vi "Test Barista Sends Pick Up Callback.vi"(8 "error in (no error)":errorcluster, 11 "Barista Test in":refnum<class "Barista Test.lvclass">) -> (0 "error out":errorcluster, 3 "Barista Test out":refnum<class "Barista Test.lvclass">)   [LabVIEW 2020, in "Barista Test.lvclass"]
uses:
  Barista Test.lvclass
  C:/Program Files (x86)/National Instruments/LabVIEW 2020/vi.lib/Astemes/LUnit/Test Case.lvclass
  Processes/People/Workers/Barista/Barista.lvclass
  C:/Program Files (x86)/National Instruments/LabVIEW 2020/vi.lib/Astemes/Triarc Framework/Process/Process.lvclass
  Support/Beverages/Beverage/Beverage.lvclass
  Test Doubles/Mock Job Handler/Mock Job Handler.lvclass
  C:/Git/astemes-triarc-examples/Coffee Shop/Processes/People/Process Job/Job Handler.lvclass
  Support/Beverages/TypeDefs/Drink Type.ctl
  Support/Beverages/TypeDefs/Options.ctl
  Support/Beverages/Beverage/Beverage.lvclass/Beverage.ctl
  <vilib>/Astemes/Triarc Framework/Process/Process.lvclass/Process.ctl
  <vilib>/Astemes/LUnit/Test Case.lvclass/Test Case.ctl
  89ef2f0c-66e7-4d1e-b839-78bb04362f4d.vi
  Support/Beverages/Beverage/Write Drink Type.vi
  Support/Beverages/Beverage/Write Options.vi
  <vilib>/Astemes/Triarc Framework/Process/Private/SubVIs/Wait for finish.vi
  <vilib>/Astemes/Triarc Framework/Process/Private/SubVIs/Set Lifecycle State.vi
  <vilib>/Astemes/Triarc Framework/Process/Protected/Messaging/Send Message.vi
  <vilib>/Astemes/Triarc Framework/Process/Public/Lifecycle/Get Lifecycle State.vi
  <vilib>/Astemes/LUnit/Palette/Pass.vi
  <vilib>/Astemes/LUnit/Palette/Fail.vi
  <vilib>/Astemes/LUnit/Compare Variants.vi
  <vilib>/Astemes/LUnit/Describe Comparison.vi
  <vilib>/Astemes/LUnit/Set Assertion Type.vi
  <vilib>/Astemes/Triarc Framework/Process/Private/SubVIs/Handle Debug Data.vi
  <vilib>/Utility/error.llb/Clear Errors.vi
  <vilib>/Astemes/LUnit/Add test result.vi
  <vilib>/Astemes/LUnit/Variant to string.vi
  <vilib>/Astemes/Triarc Framework/Logging/Log Debug.vi
  <vilib>/AdvancedString/1D String Array to Delimited String.vi
  <vilib>/Utility/High Resolution Relative Seconds.vi
  <vilib>/Astemes/LUnit/LUnit Record Assertion Result.vi
  <vilib>/Astemes/LUnit/LUnit Aggregate Assertion Results.vi
  <vilib>/Astemes/LUnit/Method Result/LUnit Merge Status.vi
  <vilib>/Astemes/LUnit/LUnit Concatenate result strings.vi
  <vilib>/Utility/error.llb/Error Cluster From Error Code.vi
  <vilib>/Astemes/Triarc Framework/Process/Public/Read Name.vi
  <vilib>/Utility/Data Type/Get Type Information.vi
  <vilib>/Utility/LVClass/Get LV Class Name.vi
  <vilib>/Astemes/Triarc Framework/Process/Process.lvclass
  Support/Order Item/Order Item.lvclass
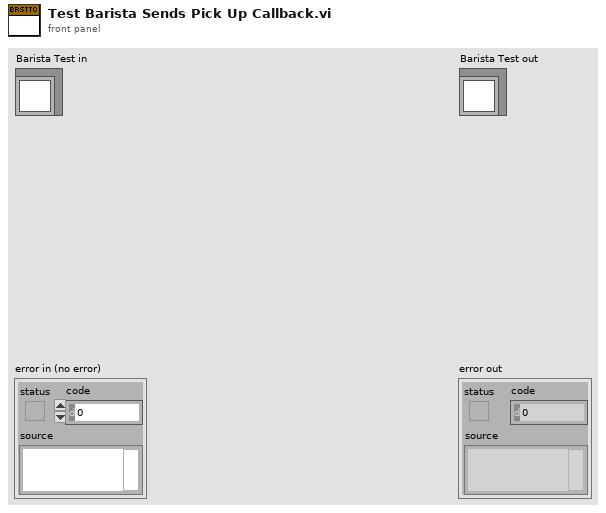
[diagram p1: front panel]
types:
  T1 = typedef "Beverage.lvclass/Options.ctl" = enum16{"<None>", "Milk", "Mocha", "Soy", "Whip"}
  T2 = typedef "Beverage.lvclass/Drink Type.ctl" = enum16{"Dark Roast", "Decaf", "Espresso", "House Blend"}
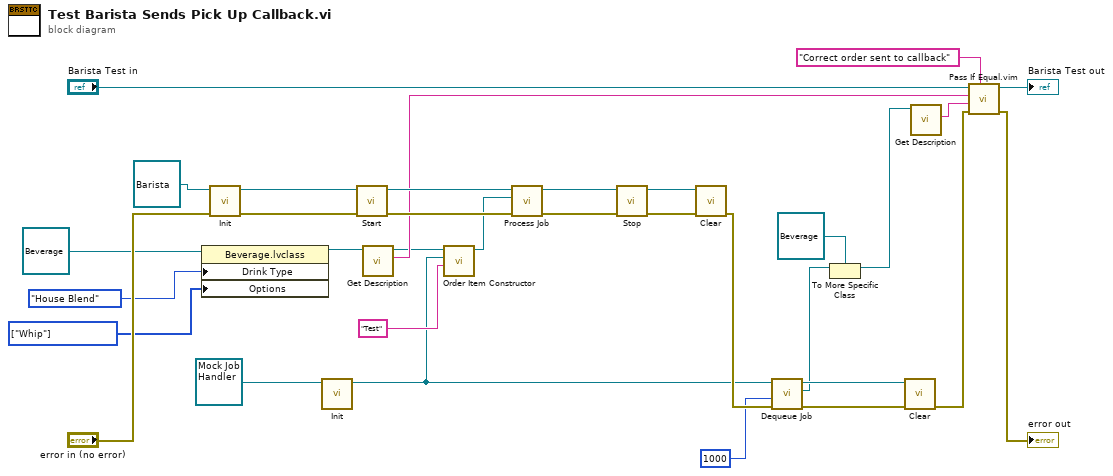
[diagram p0: block diagram]
diagram:
  w6 = T1[] [enum."Whip"] items=["<None>", "Milk", "Mocha", "Soy", "Whip"] ("Options")
  n1 = property class="Beverage.lvclass"(reference=refnum<class "Beverage.lvclass"> refnum ("Beverage"), "Drink Type"=Drink_Type."House Blend", "Options"=w6) -> (reference out=w5:refnum<class "Beverage.lvclass">)  [unwired: 1 in, 1 out]
  n2 = call-dynamic "Init.vi"("error in (no error)"="error in (no error)", "View In"=refnum<class "Barista.lvclass"> refnum ("Barista.lvclass")) -> ("error out"=w30:errorcluster, "View Out"=w26:refnum<class "Barista.lvclass">)  [unwired: 8 in]
  n3 = call-dynamic "Init.vi"("Mock Job Handler In"=refnum<class "Mock Job Handler.lvclass"> refnum ("Mock Job Handler.lvclass")) -> ("Mock Job Handler Out"=w9:refnum<class "Mock Job Handler.lvclass">)  [unwired: 9 in, 1 out]
  n4 = call <vilib>:"Start.vi"("error in (no error)"=w30, "Process In"=w26) -> ("error out"=w32:errorcluster, "Process Out"=w25:refnum<class "Barista.lvclass">)  [unwired: 7 in, 1 out]
  n5 = call "Get Description.vi"("Beverage in"=w5) -> ("Description"=w16:string, "Beverage out"=w4:refnum<class "Beverage.lvclass">)  [unwired: 8 in, 1 out]
  n6 = call "Order Item Constructor.vi"("Cust Name"="Test", "Pick Up Order Handler"=w9, "Beverage"=w4) -> ("Order Item"=w28:refnum<class "Order Item.lvclass">)  [unwired: 7 in, 1 out]
  n7 = call-dynamic "Process Job.vi"("error in (no error)"=w32, "Job"=w28, "Worker In"=w25) -> ("error out"=w22:errorcluster, "Worker Out"=w24:refnum<class "Barista.lvclass">)  [unwired: 7 in]
  n8 = call <vilib>:"Stop.vi"("error in (no error)"=w22, "Process In"=w24) -> ("error out"=w31:errorcluster, "Process Out"=w23:refnum<class "Barista.lvclass">)  [unwired: 7 in, 1 out]
  n9 = call-dynamic "Clear.vi"("error in (no error)"=w31, "View In"=w23) -> ("error out"=w20:errorcluster)  [unwired: 9 in]
  n10 = call "Dequeue Job.vi"("error in (no error)"=w20, "timeout in ms (-1)"=1000, "Mock Job Handler In"=w9) -> ("error out"=w15:errorcluster, "element"=w1:refnum<class>, "Mock Job Handler Out"=w14:refnum<class "Mock Job Handler.lvclass">)  [unwired: 5 in, 1 out]
  n11 = To More Specific Class(target class=refnum<class "Beverage.lvclass"> refnum ("Beverage out"), reference=w1) -> (specific class reference=w3:refnum<class "Beverage.lvclass">)  [unwired: 1 in, 1 out]
  n12 = call-dynamic "Clear.vi"("error in (no error)"=w15, "Mock Job Handler In"=w14) -> ("error out"=w12:errorcluster)  [unwired: 9 in]
  n13 = call "Get Description.vi"("Beverage in"=w3) -> ("Description"=w13:string)  [unwired: 8 in, 2 out]
  n14 = call "Pass If Equal.vim"("Description"="Correct order sent to callback", "error in (no error)"=w12, "Actual"=w13, "Expected"=w16, "LUnit Test Case In"="Barista Test in") -> ("error out"=→"error out":errorcluster, "LUnit Test Case Out"=→"Barista Test out":refnum<class "Barista Test.lvclass">)  [unwired: 5 in]
